vi "MeasuringDevice.Measure.vi"(8 "error in (no error)":errorcluster, 11 "OPM":refnum<class "OPM.lvclass">) -> (0 "error out":errorcluster, 2 "Result":variant, 3 "OPM out":refnum<class "OPM.lvclass">)   [LabVIEW 2019, in "OPM.lvclass"]
doc: "---------------------------------------------------------------\nJKI State Machine Objects™\nhttp://jki.net/state-machine-objects/\nCopyright (C) 2005-2015, JKI <info@jki.net>\nALL RIGHTS RESERVEDJKI State Machine Objects (SMO) 1.0.0.5\nJKI - JKI\nCopyright (c) 2016, JKI"
uses:
  OPM.lvclass
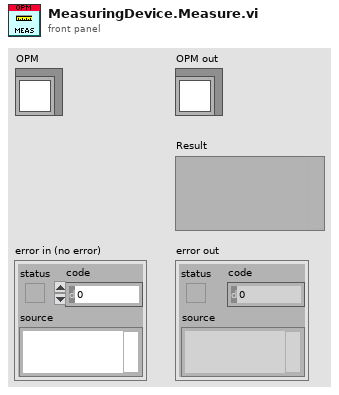
[diagram p1: front panel]
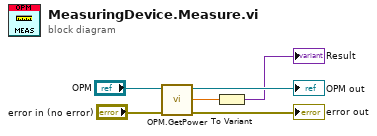
[diagram p0: block diagram]
diagram:
  n1 = call-dynamic "OPM.GetPower.vi"("error in (no error)"="error in (no error)", "PM in"="OPM") -> ("error out"=→"error out":errorcluster, "Power, W"=w3:dbl, "PM out"=→"OPM out":refnum<class "OPM.lvclass">)  [unwired: 7 in]
  n2 = To Variant(anything=w3) -> (Variant=→"Result":variant)
